vi "Extract Angle.vi"(3 "Transformation matrix":T1) -> (0 "Axis":cluster{"X":sgl, "Y":sgl, "Z":sgl}, 1 "angle":dbl)   [LabVIEW 2024]
uses:
  <vilib>/Analysis/NI_AALPro.lvlib
  <vilib>/Analysis/_algsub.llb/Real Matrix Trace.vi
  <vilib>/Analysis/_algsub.llb/Real Vector Norm.vi
  <vilib>/Analysis/Matrix/Datatypes/RealMatrix.ctl
  <vilib>/Analysis/Matrix/NI_Matrix.lvlib
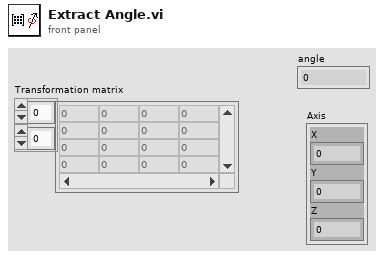
[diagram p1: front panel]
types:
  T1 = typedef "NI_Matrix.lvlib/RealMatrix.ctl" = dbl[][]
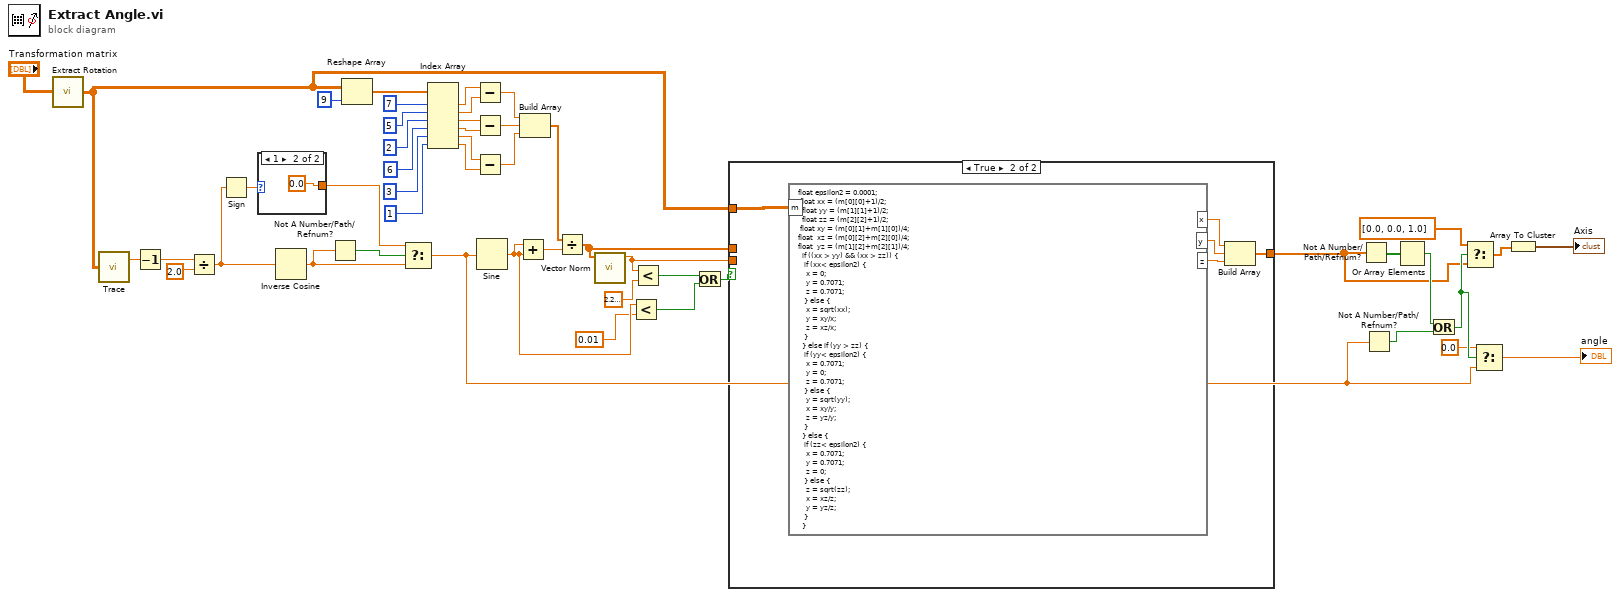
[diagram p0: block diagram]
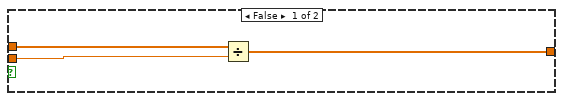
[diagram p2: hidden frame]
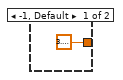
[diagram p3: hidden frame]
diagram:
  n1 = call <userlib>:"Extract Rotation.vi"("Transformation matrix"="Transformation matrix") -> ("Rotation matrix"=w2:T1)
  n2 = call-poly <vilib>:"Trace.vi"("Input Matrix"=w2) -> ("trace"=w46:dbl)  [unwired: 1 out]
  n3 = Decrement(x=w46) -> (x-1=w47:dbl)
  n4 = Divide(x=w47, y=2.0) -> (x/y=w45:dbl)
  n5 = Sign(1:w45) -> (0:w44:dbl)
  n6 = case shown="1" w44 {
    tunnel: [3.141592653589793 0.0] -> w42
    frame -1, Default {
    }
    frame 1 {
    }
  }
  n7 = Inverse Cosine(1:w45) -> (0:w41:dbl)
  n8 = Not A Number/Path/Refnum?(number/path/refnum=w41) -> (NaN/Path/Refnum?=w43:bool)
  n9 = Reshape Array(w2, 9 ("dimension size")) -> (w21:dbl[])
  n10 = Select(t=w42, s=w43, f=w41) -> (s? t:f=w5:dbl)
  n11 = Index Array(array=w21, index #1=7 ("index"), index #2=5 ("index"), index #3=2 ("index"), index #4=6 ("index"), index #5=3 ("index"), index #6=1 ("index")) -> (element #1=w33:dbl, element #2=w34:dbl, element #3=w30:dbl, element #4=w29:dbl, element #5=w32:dbl, element #6=w31:dbl)
  n12 = Subtract(x=w33, y=w34) -> (x-y=w28:dbl)
  n13 = Subtract(x=w30, y=w29) -> (x-y=w27:dbl)
  n14 = Subtract(x=w32, y=w31) -> (x-y=w26:dbl)
  n15 = Sine(x=w5) -> (sin(x)=w17:dbl)
  n16 = Add(x=w17, y=w17) -> (x+y=w25:dbl)
  n17 = Build Array(w28, w27, w26) -> (w24:dbl[])
  n18 = Divide(x=w24, y=w25) -> (x/y=w22:dbl[])
  n19 = call-poly <vilib>:"Vector Norm.vi"("Input Vector"=w22) -> ("norm"=w20:dbl)  [unwired: 9 in, 1 out]
  n20 = Less?(x=w17, y=0.01) -> (x < y?=w15:bool)
  n21 = Less?(x=w20, y=2.220446049250313e-16) -> (x < y?=w18:bool)
  n22 = Or(x=w18, y=w15) -> (x .or. y?=w14:bool)
  n23 = case shown="True" w14 {
    tunnel: w22 -> [w53 _]
    tunnel: w20 -> [w52 _]
    tunnel: [w51 w54] -> w8
    tunnel: w2 -> [_ w58]
    frame False {
      n24 = Divide(x=w53, y=w52) -> (x/y=w51:dbl[])
    }
    frame True {
      n25 = formula code="float epsilon2 = 0.0001;  \n float xx = (m[0][0]+1)/2;\n\t\tfloat yy = (m[1][1]+1)/2;\n\t\tfloat zz = (m[2][2]+1)/2;\n\tfloat\txy = (m[0][1]+m[1][0])/4;\nfloat\t\txz = (m[0][2]+m[2][0])/4;\nfloat\t\tyz = (m[1][2]+m[2][1])/4;\n\t\tif ((xx > yy) && (xx > zz)) { \n\t\t\tif (xx< epsilon2) {\n\t\t\t\tx = 0;\n\t\t\t\ty = 0.7071;\n\t\t\t\tz = 0.7071;\n\t\t\t} else {\n\t\t\t\tx = sqrt(xx);\n\t\t\t\ty = xy/x;\n\t\t\t\tz = xz/x;\n\t\t\t}\n\t\t} else if (yy > zz) {\n\t\t\tif (yy< epsilon2) {\n\t\t\t\tx = 0.7071;\n\t\t\t\ty = 0;\n\t\t\t\tz = 0.7071;\n\t\t\t} else {\n\t\t\t\ty = sqrt(yy);\n\t\t\t\tx = xy/y;\n\t\t\t\tz = yz/y;\n\t\t\t}\t\n\t\t} else {\n\t\t\tif (zz< epsilon2) {\n\t\t\t\tx = 0.7071;\n\t\t\t\ty = 0.7071;\n\t\t\t\tz = 0;\n\t\t\t} else {\n\t\t\t\tz = sqrt(zz);\n\t\t\t\tx = xz/z;\n\t\t\t\ty = yz/z;\n\t\t\t}\n\t\t}"("m"=w58) -> ("x"=w57:dbl, "y"=w56:dbl, "z"=w55:dbl)
      n26 = Build Array(w57, w56, w55) -> (w54:dbl[])
    }
  }
  n27 = Not A Number/Path/Refnum?(number/path/refnum=w8) -> (NaN/Path/Refnum?=w13:bool[])
  n28 = Not A Number/Path/Refnum?(number/path/refnum=w5) -> (NaN/Path/Refnum?=w11:bool)
  n29 = Or Array Elements(Boolean array=w13) -> (logical OR=w12:bool)
  n30 = Or(x=w12, y=w11) -> (x .or. y?=w10:bool)
  n31 = Select(t=dbl[] [0.0, 0.0, 1.0], s=w10, f=w8) -> (s? t:f=w7:dbl[])
  n32 = Select(t=0.0, s=w10, f=w5) -> (s? t:f=→"angle":dbl)
  n33 = Array To Cluster(array=w7) -> (cluster=→"Axis":cluster{"[0]":dbl, "[1]":dbl, "[2]":dbl})
